vi "Define Setpoint.vi"(7 "Channel (0: Channel A)":u16(ring) items=["Channel A", "Channel B"], 8 "error in (no error)":errorcluster, 10 "Setpoint Value":dbl, 11 "BH Druck PACE Series in":refnum<class "BH Druck PACE Series.lvclass">) -> (0 "error out":errorcluster, 2 "Setpoint Issued":dbl, 3 "BH Druck PACE Series out":refnum<class "BH Druck PACE Series.lvclass">)   [LabVIEW 2022 SP3, in "BH Druck PACE Series.lvclass"]
uses:
  BH Druck PACE Series.lvclass
  BH Druck PACE Series.lvclass/BH Druck PACE Series.ctl
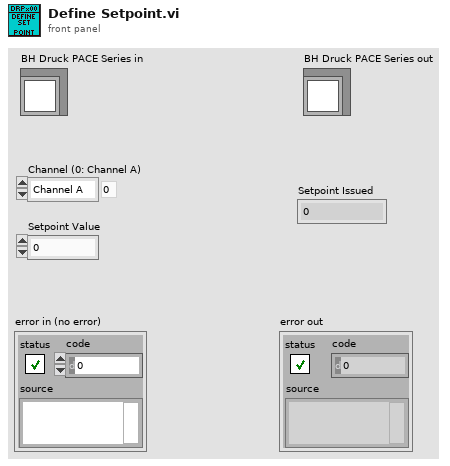
[diagram p1: front panel]
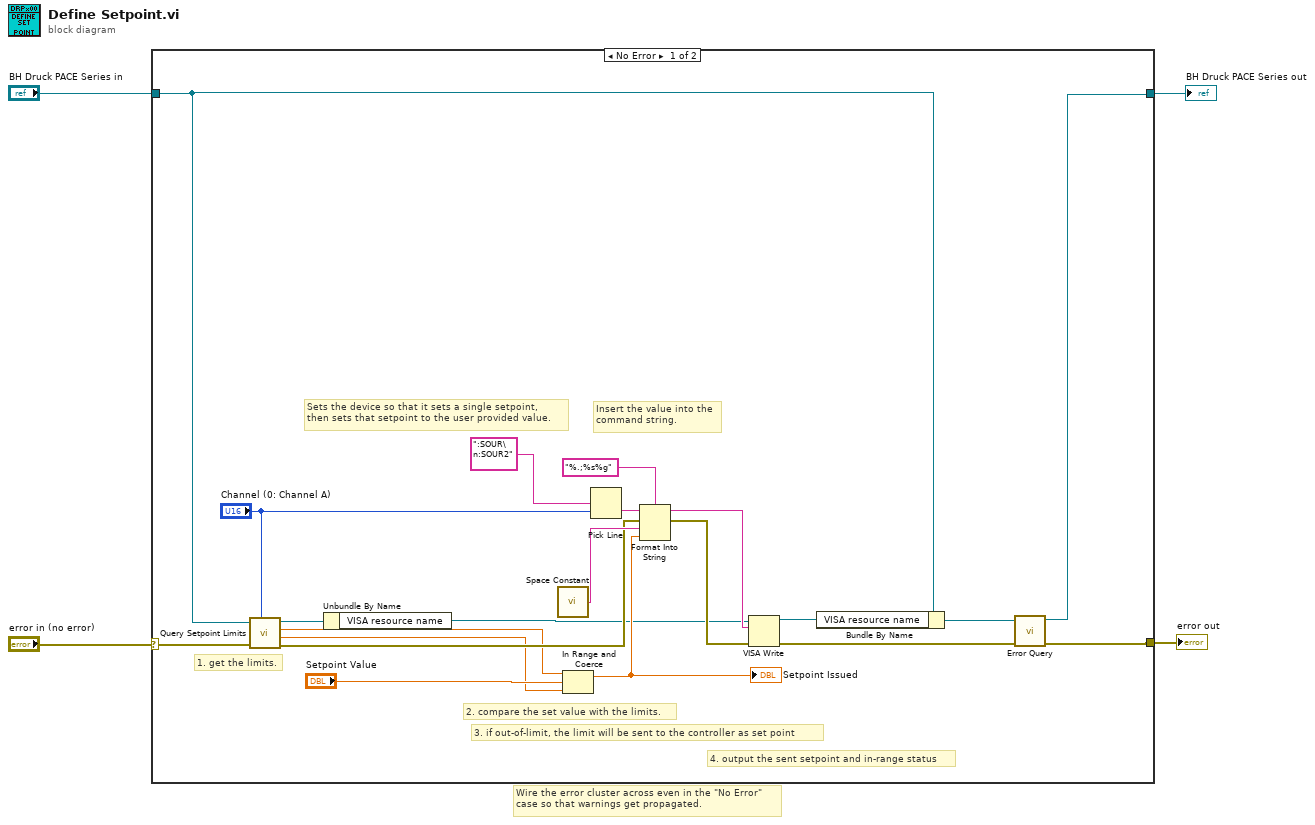
[diagram p0: block diagram]
diagram:
  # "Wire the error cluster across even in the \"No Error\"\ncase so that warnings get propagated."
  n1 = case shown="No Error" "error in (no error)" {
    selector: "error in (no error)" -> [w25 w27]
    tunnel: [w6 w27] -> w3
    tunnel: [w5 w26] -> w1
    tunnel: "BH Druck PACE Series in" -> [w11 w26]
    frame No Error {
      # "4. output the sent setpoint and in-range status"
      # "3. if out-of-limit, the limit will be sent to the controller as set point"
      # "2. compare the set value with the limits."
      # "Sets the device so that it sets a single setpoint, \nthen sets that setpoint to the user provided value."
      # "Insert the value into the\ncommand string."
      # "1. get the limits."
      n2 = call-dynamic "Query Setpoint Limits.vi"("Channel (0: Channel A)"="Channel (0: Channel A)", "error in (no error)"=w25, "BH Druck PACE Series in"=w11) -> ("error out"=w17:errorcluster, "Lower Setpoint Limit"=w14:dbl, "Upper Setpoint Limit"=w15:dbl, "BH Druck PACE Series out"=w13:refnum<class "BH Druck PACE Series.lvclass">)  [unwired: 5 in]
      n3 = Unbundle By Name(w13) -> ("VISA resource name"=w12:refnum<visa-resource-name>)
      n4 = call <vilib>:"Space Constant.vi"() -> ("String"=w21:string)
      n5 = In Range and Coerce(upper limit=w15, x="Setpoint Value", lower limit=w14) -> (coerced(x)=w19:dbl)  [unwired: 1 out]
      "Setpoint Issued" <- w19
      n6 = Pick Line(multi-line string=":SOUR\n:SOUR2", line index="Channel (0: Channel A)") -> (output string=w24:string)  [unwired: 1 in]
      n7 = Format Into String(format string="%.;%s%g", initial string=w24, error in=w17, w21, w19) -> (resulting string=w23:string, error out=w22:errorcluster)
      n8 = VISA Write(VISA resource name=w12, write buffer=w23, error in (no error)=w22) -> (VISA resource name out=w10:refnum<visa-resource-name>, error out=w8:errorcluster)  [unwired: 1 out]
      n9 = Bundle By Name(cluster=w11, "VISA resource name"=w10) -> (w7:refnum<class "BH Druck PACE Series.lvclass">)
      n10 = call-dynamic "Error Query.vi"("error in (no error)"=w8, "BH Druck PACE Series in"=w7) -> ("error out"=w6:errorcluster, "BH Druck PACE Series out"=w5:refnum<class "BH Druck PACE Series.lvclass">)  [unwired: 8 in]
    }
    frame Error {
    }
  }
  "error out" <- w3
  "BH Druck PACE Series out" <- w1
